vi "ToString.vi"(8 "error in (no error)":errorcluster, 11 "Is Less Than in":refnum<class "Is Less Than.lvclass">) -> (0 "error out":errorcluster, 2 "String":string, 3 "Is Less Than out":refnum<class "Is Less Than.lvclass">)   [LabVIEW 2017, in "Transparent Assertions.lvlib" / "Constraints.lvlib" / "Is Less Than.lvclass"]
doc: "Returns a string representation of the object."
uses:
  Is Less Than.lvclass
  Is Less Than.lvclass/Is Less Than.ctl
  5530d5e5-524e-4b10-a38f-b2ce1f8e1ddc.vi
  5530d5e5-524e-4b10-a38f-b2ce1f8e1ddc.vi/44b1e8a8-a959-4404-89ed-6e884ef6f19a.vi
  <vilib>/PNR/JSONtext Object Serialization/Generic Object Serializer/Generic Object Serializer.lvclass
  C:/Program Files/National Instruments/LabVIEW 2017/vi.lib/JDP Science/JSONtext/LVClass Serializer/JSONtext LVClass Serializer.lvclass
  <vilib>/JDP Science/JSONtext/Variant to JSON Text.vi
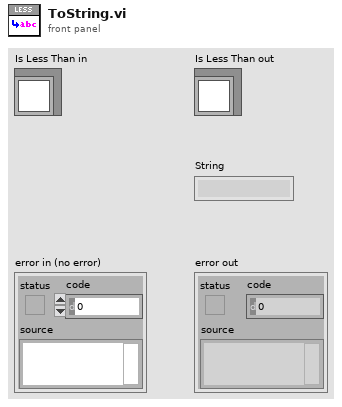
[diagram p1: front panel]
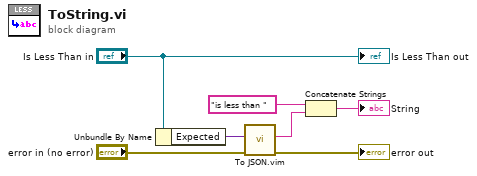
[diagram p0: block diagram]
diagram:
  n1 = Unbundle By Name("Is Less Than in") -> ("Expected"=w4:variant)
  n2 = call "To JSON.vim"("error in (no error)"="error in (no error)", "Anything"=w4) -> ("error out"=→"error out":errorcluster, "JSON"=w2:string)  [unwired: 8 in]
  n3 = Concatenate Strings("is less than " ("String"), w2) -> (→"String":string)
  "Is Less Than out" <- "Is Less Than in"
